vi "Setup.vi"(0 "Ramper.in":refnum<class "Ramper.lvclass">, 1 "Ramp control refnum":refnum<vi>, 2 "Parameter":dbl, 3 "Upper Limit":dbl, 5 "Ramp rate":dbl, 7 "Min increment":dbl, 9 "Formula":string, 11 "error in (no error)":errorcluster, 14 "Lower limit":dbl) -> (4 "Ramper.out":refnum<class "Ramper.lvclass">, 15 "error out":errorcluster)   [LabVIEW 2014, in "Ramper.lvclass"]
uses:
  Ramper.lvclass
  Ramper.lvclass/Ramper.ctl
  <vilib>/gmath/NI_Gmath.lvlib
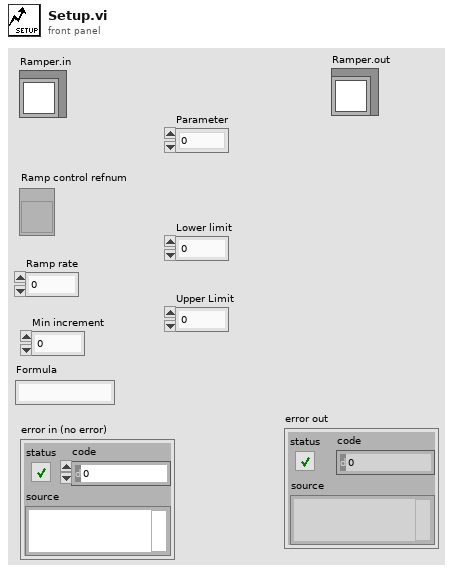
[diagram p1: front panel]
types:
  T1 = cluster{"Y Values":dbl[][], "Tables":i32[][][], "Variables input decode":i32[], "Variables output decode":i32[]}
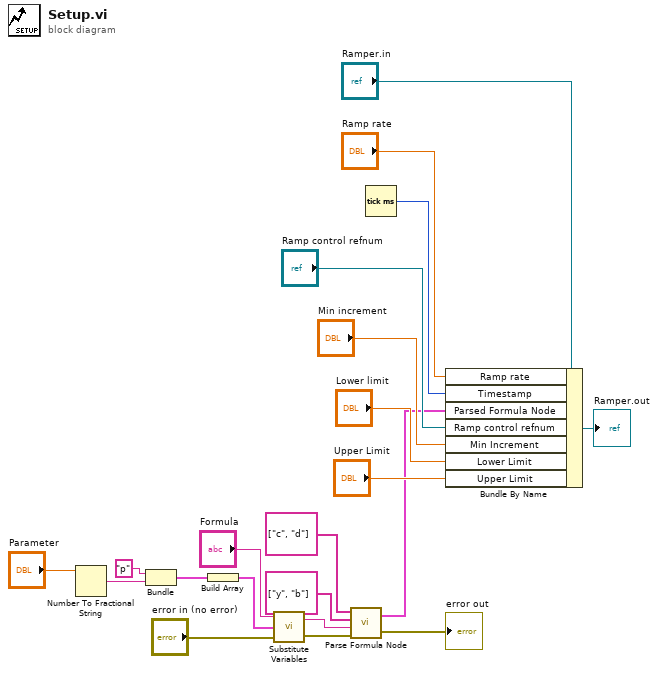
[diagram p0: block diagram]
diagram:
  n1 = Number To Fractional String(number="Parameter") -> (F-format string=w12:string)  [unwired: 3 in]
  n2 = Bundle("p", w12) -> (w11:cluster{string, string})  [unwired: 1 in]
  n3 = Build Array(w11) -> (w10:cluster{string, string}[])
  n4 = call <vilib>:"Substitute Variables.vi"("error in (no error)"="error in (no error)", "Substitution Rules"=w10, "original formula"="Formula") -> ("error out"=w5:errorcluster, "formula after substitution"=w6:string)
  n5 = call <vilib>:"Parse Formula Node.vi"("error in (no error)"=w5, "formula"=w6, "Variables Output"=string[] ["y", "b"], "Variables Input"=string[] ["c", "d"]) -> ("error out"=→"error out":errorcluster, "Parsed Formula Node"=w1:T1)
  n6 = Tick Count (ms)() -> (millisecond timer value=w18:u32)
  n7 = Bundle By Name(cluster="Ramper.in", "Ramp rate"="Ramp rate", "Timestamp"=w18, "Parsed Formula Node"=w1, "Ramp control refnum"="Ramp control refnum", "Min Increment"="Min increment", "Lower Limit"="Lower limit", "Upper Limit"="Upper Limit") -> (→"Ramper.out":refnum<class "Ramper.lvclass">)
